vi "DSF.Shared.Configuration.Transfer Group.Load from Disk.vi"(8 "error in (no error)":errorcluster, 10 "object":refnum<class>, 11 "Transfer Group Configuration in":refnum<class "DSF.Shared.Configuration.Transfer Group.lvclass">) -> (0 "error out":errorcluster, 3 "Transfer Group Configuration out":refnum<class "DSF.Shared.Configuration.Transfer Group.lvclass">)   [LabVIEW 2016, in "DSF.Shared.lvlib" / "DSF.Shared.Configuration.Transfer Group.lvclass"]
uses:
  DSF.Shared.Configuration.Transfer Group.lvclass
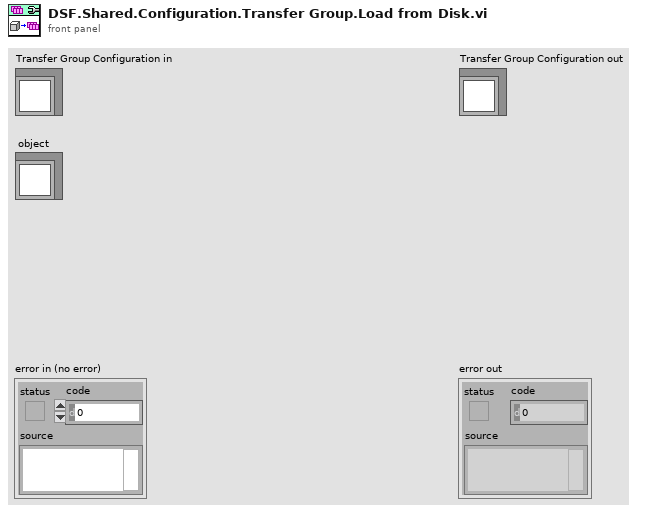
[diagram p1: front panel]
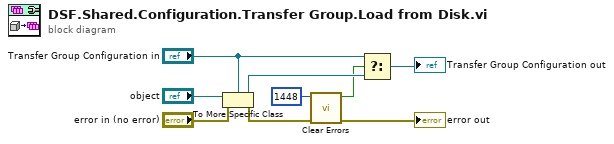
[diagram p0: block diagram]
diagram:
  n1 = To More Specific Class(target class="Transfer Group Configuration in", reference="object", error in="error in (no error)") -> (specific class reference=w7:refnum<class "DSF.Shared.Configuration.Transfer Group.lvclass">, error out=w8:errorcluster)
  n2 = call <vilib>:"Clear Errors.vi"("error in (no error)"=w8, "specific error code to clear (0: all)"=1448) -> ("error out"=→"error out":errorcluster, "specific error cleared?"=w6:bool)  [unwired: 4 in]
  n3 = Select(t="Transfer Group Configuration in", s=w6, f=w7) -> (s? t:f=→"Transfer Group Configuration out":refnum<class "DSF.Shared.Configuration.Transfer Group.lvclass">)
